vi "test_HLAfloat64BE.vi"() -> ()   [LabVIEW 2019, in "HLA Data Conversion.lvlib"]
uses:
  HLA Data Conversion.lvlib
panel:
  out "eu data out":dbl[](array[numeric])
  out "valid 2":bool=TRUE
  out "valid":bool=TRUE
  in  "eu data in":dbl[](array[numeric])=[2.3456]
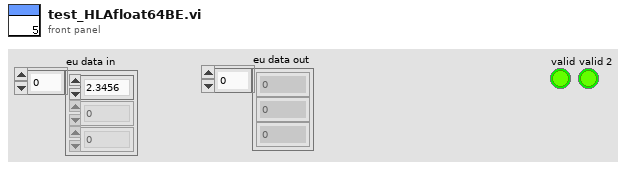
[diagram p1: front panel]
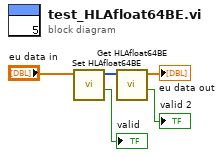
[diagram p0: block diagram]
diagram:
  n1 = call "Set HLAfloat64BE.vi"("eu data in"="eu data in") -> ("valid"=→"valid":bool, "raw data out"=w5:u8[])  [unwired: 9 in]
  n2 = call "Get HLAfloat64BE.vi"("raw data in"=w5) -> ("valid"=→"valid 2":bool, "eu data out"=→"eu data out":dbl[])  [unwired: 9 in]
